vi "Module Loop.vi"(8 "error in (no error)":errorcluster, 11 "Sequencing in":refnum<class "Sequencing.lvclass">) -> (0 "error out":errorcluster, 3 "Sequencing out":refnum<class "Sequencing.lvclass">)   [LabVIEW 2020, in "VolatusSeq.lvlib" / "Sequencing.lvclass"]
uses:
  Sequencing.lvclass
  C:/dev/lv20CE/relink/lv-volatus/Volatus/Module/Module.lvclass
  Volatus/Module/Module.lvclass/Module.ctl
  Volatus/MessageQ/MessageQ.lvclass/MessageQ.ctl
  Sequencing.lvclass/Sequencing.ctl
  Volatus/Module/Module.lvclass
  Sequence Load Data.ctl
  lv-promises/Promises/Value/Value.lvclass
  Sequence Status.ctl
  Sequence Time.ctl
  Sequence Status Value/Sequence Status Value.lvclass/Sequence Status Value.ctl
  Sequence/Sequence.lvclass/Sequence.ctl
  Sequencing Status Value/Sequencing Status Value.lvclass/Sequencing Status Value.ctl
  lv-web-crypto/lv-crypto/Crypto/Hashes/SHA-256/SHA-256.lvclass
  d0d387a8-945a-4f27-bd1a-8c3fe56f864d.vi
  f3a44cdb-5a36-43f0-b83a-6d3fbfdadde6.vi
  31a4c29e-fb87-4ad3-ba8b-3d056e126c3f.vi
  93d0e60a-9556-42ac-a023-1725ae64f642.vi
  <vilib>/JDP Science/JSONtext/Next JSON Value.vi
  <vilib>/JDP Science/JSONtext/String Subset.vi
  Sequence/CRC.vi
  <vilib>/JDP Science/JSONtext/Parsing/Advance past next JSON Value (inlined COPY).vi
  <vilib>/JDP Science/JSONtext/Parsing/Advance past whitespace.vi
  <vilib>/JDP Science/JSONtext/Parsing/Advance past String.vi
  <vilib>/JDP Science/JSONtext/Parsing/Advance past Number.vi
  <vilib>/JDP Science/JSONtext/Parsing/Advance past Line Ending.vi
  <vilib>/JDP Science/JSONtext/Parsing/Parse Full Path or Item Name.vi
  <vilib>/JDP Science/JSONtext/Parsing/Advance past Array.vi
  <vilib>/JDP Science/JSONtext/Parsing/Advance past Object.vi
  <vilib>/JDP Science/JSONtext/support/Error Cluster From Code.vi
  <vilib>/JDP Science/JSONtext/Offset/Find Item Locations by Path.vi
  <vilib>/JDP Science/JSONtext/JSON text to Variant.vi
  <vilib>/JDP Science/JSONtext/LVClass Serializer/JSONtext LVClass Serializer.lvclass
  Sequence/Sequence.lvclass
  lv-promises/Promises/Promise/Promise.lvclass
  Sequence Status Value/Sequence Status Value.lvclass
  Sequencing Status Value/Sequencing Status Value.lvclass
  VolatusSeq.lvlib
  Volatus/MessageQ/MessageQ.lvclass
  <vilib>/JDP Science/JSONtext/JSONtext.lvlib
  lv-web-crypto/lv-crypto/Crypto/Crypto.lvlib
  C:/dev/lv20CE/relink/lv-volatus/VolatusSeq/Sequencing/Sequencing.lvclass
panel:
  out "Depth":i32
  in  "Abort":bool
  in  "Unload":bool
  in  "Start":bool
  in  "Load":bool
  in  "VSEQ":string="{\n    \"Sequence\": {\n        \"Name\": \"Bottle Condition\",\n        \"Version\": \"1\",\n        \"Comment\": \"Control state machine for bottle heating/cooling.\",\n        \"Entry\": \"Start\",\n        \"Abort\": \"Stop\",\n        \"States\": {\n            \"Start\": {\n                \"Comment\": \"Reset bottle controls to off state.\",\n                \"Steps\": [\n                    {\n                        \"Time\": 0,\n                        \"Commands\": [\n                            {\"Type\": \"Transition\", \"Target\": \"Hold\"}\n                        ]\n                    }\n                ]\n            },\n            \"Hold\": {\n                \"Comment\": \"Bottle in range, controls off.\",\n                \"Steps\": [\n                    {\n                        \"Time\": 0,\n                        \"Commands\": [\n                            {\"Type\": \"Digital\", \"Channel\": \"BottleCool\", \"Value\": false},\n                            {\"Type\": \"Digital\", \"Channel\": \"BottleHeat\", \"Value\": false}\n                        ]\n                    }\n                ],\n                \"Transitions\": [\n                    {\n                        \"Type\": \"State\",\n                        \"Target\": \"Cool\",\n                        \"Logic\": \"Any\",\n                        \"Conditions\": [\n                            {\"Type\": \"HighLimit\", \"Channel\": \"BottlePSI\", \"Limit\": 850}\n                        ]\n                    },\n                    {\n                        \"Type\": \"State\",\n                        \"Target\": \"Heat\",\n                        \"Logic\": \"Any\",\n                        \"Conditions\": [\n                            {\"Type\": \"LowLimit\", \"Channel\": \"BottlePSI\", \"Limit\": 750}\n                        ]\n                    }\n                ]\n            },\n            \"Cool\": {\n                \"Comment\": \"Cooling, wait for pressure to drop.\",\n                \"Steps\": [\n                    {\n                        \"Time\": 0,\n                        \"Commands\": [\n                            {\"Type\": \"Digital\", \"Channel\": \"BottleCool\", \"Value\": true}\n                        ]\n                    }\n                ],\n                \"Transitions\": [\n                    {\n                        \"Type\": \"State\",\n                        \"Target\": \"Start\",\n                        \"Logic\": \"Any\",\n                        \"Conditions\": [\n                            {\"Type\": \"LowLimit\", \"Channel\": \"BottlePSI\", \"Limit\": 800}\n                        ]\n                    }\n                ]\n            },\n            \"Heat\": {\n                \"Comment\": \"Heating, wait for pressure to rise.\",\n                \"Steps\": [\n                    {\n                        \"Time\": 0,\n                        \"Commands\": [\n                            {\"Type\": \"Digital\", \"Channel\": \"BottleHeat\", \"Value\": true}\n                        ]\n                    }\n                ],\n                \"Transitions\": [\n                    {\n                        \"Type\": \"State\",\n                        \"Target\": \"Start\",\n                        \"Logic\": \"Any\",\n                        \"Conditions\": [\n                            {\"Type\": \"HighLimit\", \"Channel\": \"BottlePSI\", \"Limit\": 800}\n                        ]\n                    }\n                ]\n            },\n            \"Stop\": {\n                \"Comment\": \"Stopping, ensure controls off.\",\n                \"Steps\": [\n                    {\n                        \"Time\": 0,\n                        \"Commands\": [\n                            {\"Type\": \"Digital\", \"Channel\": \"BottleCool\", \"Value\": false},\n                            {\"Type\": \"Digital\", \"Channel\": \"BottleHeat\", \"Value\": false}\n                        ]\n                    }\n                ]\n            }\n        }\n    }\n}"
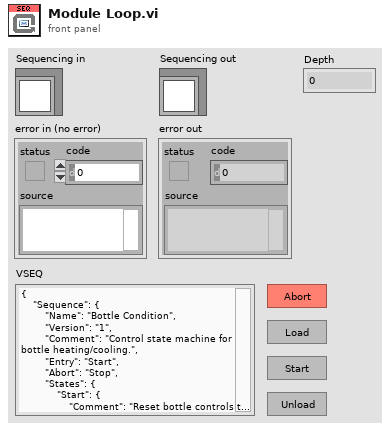
[diagram p1: front panel]
types:
  T1 = typedef "VolatusSeq.lvlib/Sequence Load Data.ctl" = cluster{"Name":string, "JSON":string, "Hash":string}
  T2 = enum32{"Invalid", "Standard", "Closed", "Hidden", "Minimized", "Maximized"}
  T3 = typedef "VolatusSeq.lvlib/Sequence Status.ctl" = cluster{"Name":string, "State":string, "Time":T4, "Running":bool, "Start Time":dbl, "Previous Duration":i64, "Previous Late":bool}
  T4 = typedef "VolatusSeq.lvlib/Sequence Time.ctl" = cluster{"Abort":bool, "Seq Time":dbl, "State Time":dbl, "Wall Time":dbl}
  T5 = typedef "VolatusSeq.lvlib/Sequencing Status.ctl" = cluster{"Sequences":T6[]}
  T6 = typedef "VolatusSeq.lvlib/Sequence Status Extended.ctl" = cluster{"Status":T3, "Loaded":bool, "CRC32":u32, "BG Color":string, "error":errorcluster}
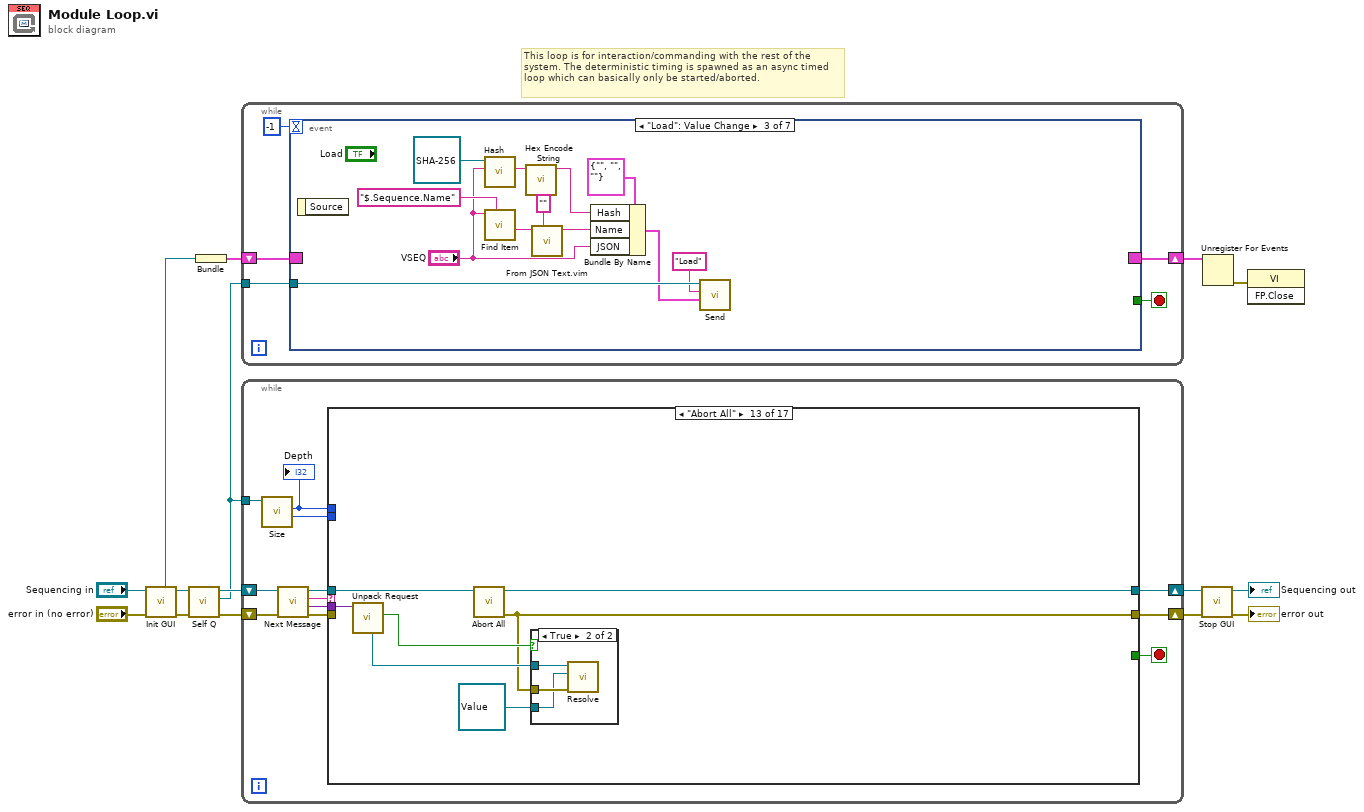
[diagram p0: block diagram]
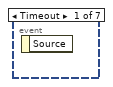
[diagram p2: hidden frame]
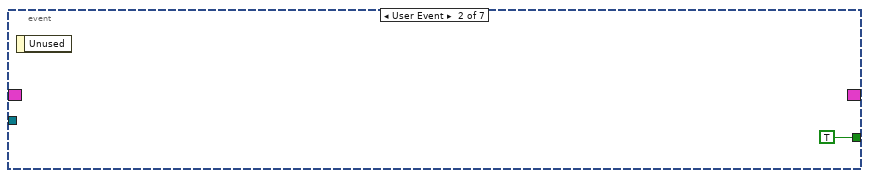
[diagram p3: hidden frame]
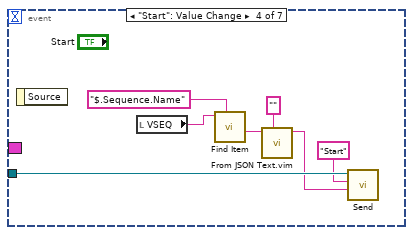
[diagram p4: hidden frame]
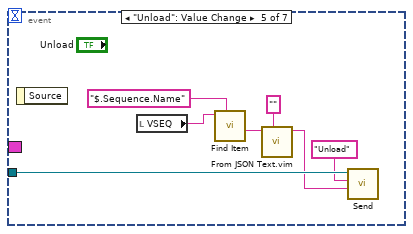
[diagram p5: hidden frame]
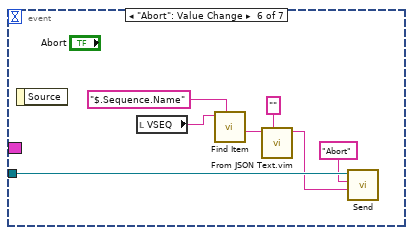
[diagram p6: hidden frame]
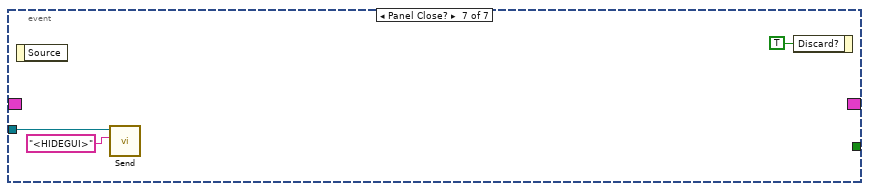
[diagram p7: hidden frame]
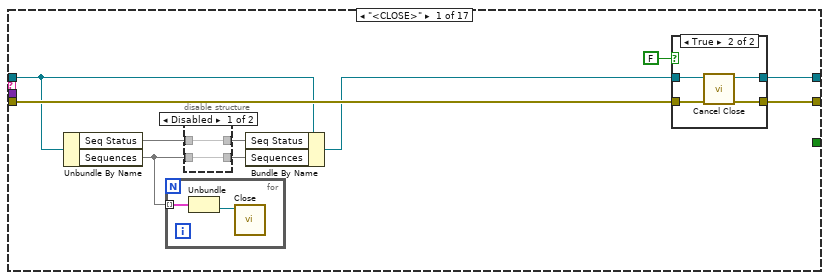
[diagram p8: hidden frame]
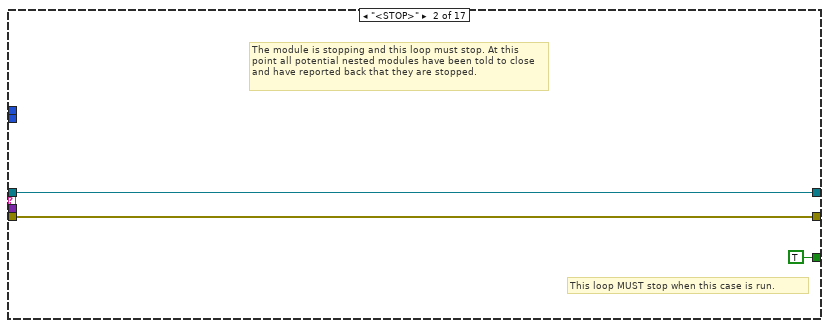
[diagram p11: hidden frame]
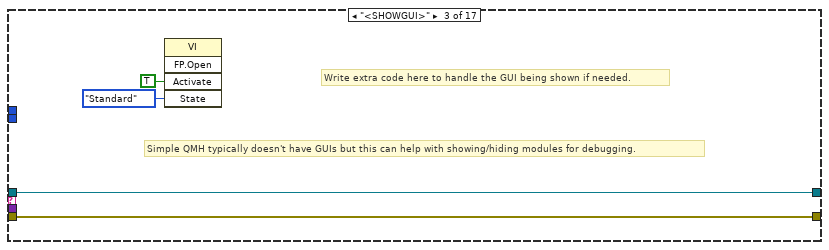
[diagram p12: hidden frame]
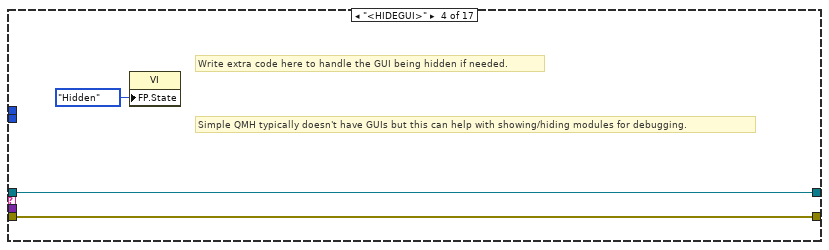
[diagram p13: hidden frame]
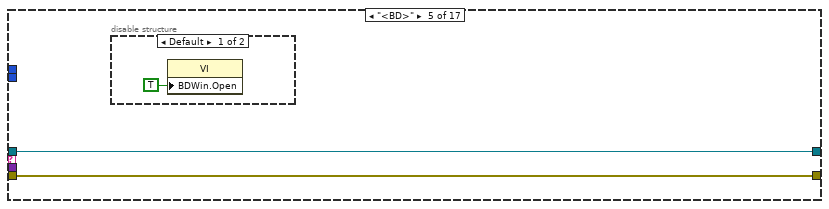
[diagram p14: hidden frame]
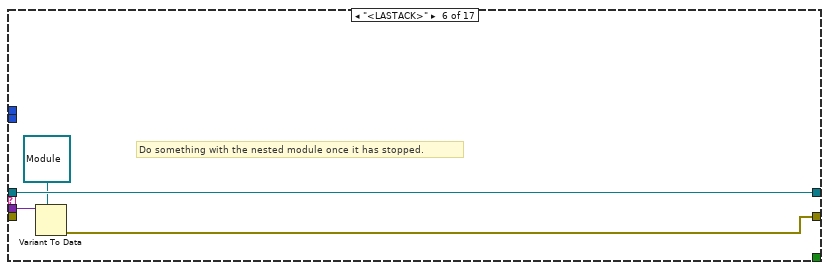
[diagram p16: hidden frame]
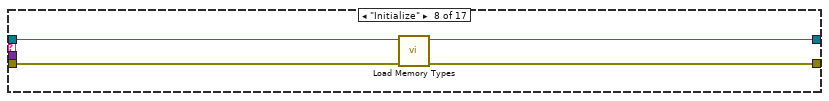
[diagram p18: hidden frame]
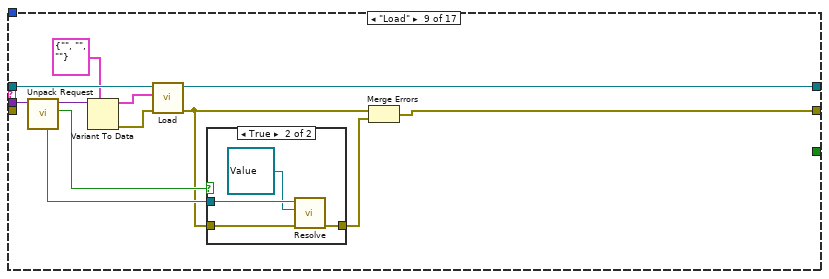
[diagram p19: hidden frame]
diagram:
  # "This loop is for interaction/commanding with the rest of the system. The deterministic timing is spawned as an async timed loop which can basically only be started/aborted."
  n1 = call "Init GUI.vi"("Module in"="Sequencing in") -> ("Module out"=w12:refnum<class "Sequencing.lvclass">, "Event Reg"=w10:refnum<event-registration>)  [unwired: 9 in]
  n2 = call "Self Q.vi"("Module in"=w12) -> ("Self Q"=w1:refnum<class "MessageQ.lvclass">, "Module out"=w8:refnum<class "Sequencing.lvclass">)  [unwired: 9 in]
  n3 = Bundle("Event Reg"=w10) -> (w11:cluster{"Event Reg":refnum<event-registration>})  [unwired: 1 in]
  n4 = while {
    tunnel: w1 -> [w18]
    shift-right: [w16] -> w4
    shift-left: w11 -> [w17]
    stop <- w15 stop-if-true
    n5 = event shown="[2] \"Load\": Value Change" {
      selector: w17 -> [_ _ _ _ _ _ _]
      dyn-events: [_ _ _ _ _ _ _] -> w16
      timeout: -1 -> [_ _ _ _ _ _ _]
      tunnel: w18 -> [_ _ w23 w34 w41 w48 w54]
      tunnel: [_ TRUE _ _ _ _ _] -> w15
      event Timeout {
        n6 = event-data() -> ()  [unwired: 1 in, 1 out]
      }
      event User Event {
        n7 = event-data() -> ()  [unwired: 1 in, 1 out]
      }
      event "Load": Value Change {
        n8 = event-data() -> ()  [unwired: 1 in, 1 out]
        n9 = call-dynamic "Hash.vi"("Message"="VSEQ", "SHA-256 in"=refnum<class "SHA-256.lvclass"> refnum) -> ("Hash"=w25:string)  [unwired: 7 in, 2 out]
        n10 = call <vilib>:"Find Item.vi"("$Path or Item Name"="$.Sequence.Name", "JSON"="VSEQ") -> ("<JSON>"=w30:string)  [unwired: 6 in, 3 out]
        n11 = call "Hex Encode String.vi"("String"=w25) -> ("Hex Encoded String"=w20:string)  [unwired: 10 in]
        n12 = call "From JSON Text.vim"("Data Type and Default Value"="", "JSON"=w30) -> ("Data out"=w26:string)  [unwired: 8 in, 1 out]
        n13 = Bundle By Name(cluster=T1 {"Name"="", "JSON"="", "Hash"=""} ("Sequence Load Data"), "Hash"=w20, "Name"=w26, "JSON"="VSEQ") -> (w22:T1)
        n14 = call "Send.vi"("Data"=w22, "ID"="Load", "MessageQ in"=w23) -> ()  [unwired: 7 in, 2 out]
      }
      event "Start": Value Change {
        n15 = event-data() -> ()  [unwired: 1 in, 1 out]
        n16 = local read "VSEQ"() -> (w35:string)
        n17 = call <vilib>:"Find Item.vi"("$Path or Item Name"="$.Sequence.Name", "JSON"=w35) -> ("<JSON>"=w37:string)  [unwired: 6 in, 3 out]
        n18 = call "From JSON Text.vim"("Data Type and Default Value"="", "JSON"=w37) -> ("Data out"=w33:string)  [unwired: 8 in, 1 out]
        n19 = call "Send.vi"("Data"=w33, "ID"="Start", "MessageQ in"=w34) -> ()  [unwired: 7 in, 2 out]
      }
      event "Unload": Value Change {
        n20 = event-data() -> ()  [unwired: 1 in, 1 out]
        n21 = local read "VSEQ"() -> (w42:string)
        n22 = call <vilib>:"Find Item.vi"("$Path or Item Name"="$.Sequence.Name", "JSON"=w42) -> ("<JSON>"=w44:string)  [unwired: 6 in, 3 out]
        n23 = call "From JSON Text.vim"("Data Type and Default Value"="", "JSON"=w44) -> ("Data out"=w40:string)  [unwired: 8 in, 1 out]
        n24 = call "Send.vi"("Data"=w40, "ID"="Unload", "MessageQ in"=w41) -> ()  [unwired: 7 in, 2 out]
      }
      event "Abort": Value Change {
        n25 = event-data() -> ()  [unwired: 1 in, 1 out]
        n26 = local read "VSEQ"() -> (w49:string)
        n27 = call <vilib>:"Find Item.vi"("$Path or Item Name"="$.Sequence.Name", "JSON"=w49) -> ("<JSON>"=w51:string)  [unwired: 6 in, 3 out]
        n28 = call "From JSON Text.vim"("Data Type and Default Value"="", "JSON"=w51) -> ("Data out"=w47:string)  [unwired: 8 in, 1 out]
        n29 = call "Send.vi"("Data"=w47, "ID"="Abort", "MessageQ in"=w48) -> ()  [unwired: 7 in, 2 out]
      }
      event Panel Close? {
        n30 = event-data() -> ()  [unwired: 1 in, 1 out]
        n31 = call "Send.vi"("ID"="<HIDEGUI>", "MessageQ in"=w54) -> ()  [unwired: 8 in, 2 out]
        n32 = event-data("Discard?"=TRUE) -> ()  [unwired: 1 in, 1 out]
      }
    }
  }
  n33 = while {
    shift-right: [w62] -> w5
    shift-left: w8 -> [w67]
    shift-right: [w61] -> w6
    shift-left: "error in (no error)" -> [w66]
    tunnel: w1 -> [w58]
    stop <- w60 stop-if-true
    n34 = call "Size.vi"("MessageQ in"=w58) -> ("Max Size"=w56:i32, "Depth"=w57:i32)  [unwired: 7 in, 2 out]
    "Depth" <- w57
    n35 = call "Next Message.vi"("error in (no error)"=w66, "Module in"=w67) -> ("error out"=w65:errorcluster, "Data"=w59:variant, "ID"=w64:string, "Module out"=w63:refnum<class "Sequencing.lvclass">)  [unwired: 6 in]
    n36 = case shown="\"Abort All\"" w64 {
      tunnel: w65 -> [w77 w89 w93 w96 w98 _ w105 w110 _ _ _ _ _ _ _ _ w231]
      tunnel: w63 -> [w70 w90 w94 w97 w99 w104 w106 w108 w122 w134 w148 w162 w174 w183 w207 w226 w229]
      tunnel: [w75 w90 w94 w97 w99 w104 w106 w107 w118 w133 w147 w161 w173 w181 w207 w225 w228] -> w62
      tunnel: [w76 w89 w93 w96 w98 w101 w105 w109 w111 w127 w141 w155 w169 w179 w201 w220 w230] -> w61
      tunnel: [_ TRUE _ _ _ _ _ _ _ _ _ _ _ _ _ _ _] -> w60
      tunnel: w59 -> [_ _ _ _ _ w103 _ _ w121 w137 w151 w165 w175 w185 w210 w224 _]
      tunnel: w57 -> [_ _ _ _ _ _ _ _ _ _ _ _ _ _ _ _ _]
      tunnel: w56 -> [_ _ _ _ _ _ _ _ _ _ _ _ _ _ _ _ _]
      frame "<CLOSE>" {
        n37 = Unbundle By Name(w70) -> ("Seq Status"=w68:map{string, T3}, "Sequences"=w73:map{string, refnum<class "Sequence.lvclass">})
        n38 = for {
          tunnel: w73 -> [w81] mode=indexing
          n39 = Unbundle(w81) -> ("Sequence"=w80:refnum<class "Sequence.lvclass">)  [unwired: 1 out]
          n40 = call "Close.vi"("Sequence in"=w80) -> ()  [unwired: 9 in, 2 out]
        }
        n41 = disable-structure shown="Disabled" {
          disable-tunnel: w73 -> [w79 _]
          disable-tunnel: [w79 _] -> w72
          disable-tunnel: [w78 _] -> w69
          disable-tunnel: w68 -> [w78 _]
          frame Disabled {
          }
          frame Enabled {
          }
        }
        n42 = Bundle By Name(cluster=w70, "Seq Status"=w69, "Sequences"=w72) -> (w71:refnum<class "Sequencing.lvclass">)
        n43 = case shown="True" FALSE {
          tunnel: w77 -> [w82 w87]
          tunnel: [w82 w86] -> w76
          tunnel: w71 -> [w83 w85]
          tunnel: [w83 w84] -> w75
          frame False {
          }
          frame True {
            n44 = call "Cancel Close.vi"("error in (no error)"=w87, "Module in"=w85) -> ("error out"=w86:errorcluster, "Module out"=w84:refnum<class "Sequencing.lvclass">)  [unwired: 8 in]
          }
        }
      }
      frame "<STOP>" {
        # "This loop MUST stop when this case is run."
        # "The module is stopping and this loop must stop. At this point all potential nested modules have been told to close and have reported back that they are stopped."
      }
      frame "<SHOWGUI>" {
        # "Simple QMH typically doesn't have GUIs but this can help with showing/hiding modules for debugging."
        # "Write extra code here to handle the GUI being shown if needed."
        n45 = invoke class="VI" method="FP.Open"("Activate"=TRUE ("Activate?"), "State"=T2."Standard") -> ()  [unwired: 3 in, 5 out]
      }
      frame "<HIDEGUI>" {
        # "Simple QMH typically doesn't have GUIs but this can help with showing/hiding modules for debugging."
        # "Write extra code here to handle the GUI being hidden if needed."
        n46 = property class="VI"("FP.State"=T2."Hidden" ("Front Panel Window:State")) -> ()  [unwired: 2 in, 2 out]
      }
      frame "<BD>" {
        n47 = disable-structure shown="Default" {
          frame condition #0 (active) {
            n48 = property class="VI"("BDWin.Open"=TRUE ("Block Diagram Window:Open")) -> ()  [unwired: 2 in, 2 out]
          }
          frame condition #1 {
          }
        }
      }
      frame "<LASTACK>" {
        # "Do something with the nested module once it has stopped."
        n49 = Variant To Data(type=refnum<class "Module.lvclass"> refnum ("Volatus:Module"), Variant=w103) -> (error out=w101:errorcluster)  [unwired: 1 in, 1 out]
      }
      frame "<TIMEOUT>" {
      }
      frame "Initialize" {
        n50 = call "Load Memory Types.vi"("error in (no error)"=w110, "Sequencing in"=w108) -> ("error out"=w109:errorcluster, "Sequencing out"=w107:refnum<class "Sequencing.lvclass">)  [unwired: 8 in]
      }
      frame "Load" {
        n51 = call "Unpack Request.vi"("Request Data"=w121) -> ("Is Request"=w115:bool, "Data"=w120:variant, "Promise"=w114:refnum<class "Promise.lvclass">)  [unwired: 8 in]
        n52 = Variant To Data(type=T1 {"Name"="", "JSON"="", "Hash"=""} ("Sequence Load Data"), Variant=w120) -> (data=w117:T1, error out=w116:errorcluster)  [unwired: 1 in]
        n53 = call "Load.vi"("error in (no error)"=w116, "Sequence Load Data"=w117, "Sequencing in"=w122) -> ("error out"=w113:errorcluster, "Sequencing out"=w118:refnum<class "Sequencing.lvclass">)  [unwired: 7 in]
        n54 = case shown="True" w115 {
          tunnel: w114 -> [_ w126]
          tunnel: w113 -> [_ w125]
          tunnel: [_ w124] -> w112
          frame False {
          }
          frame True {
            n55 = call "Resolve.vi"("error in (no error)"=w125, "Result (None)"=refnum<class "Value.lvclass"> refnum ("Result"), "Promise in"=w126) -> ("error out"=w124:errorcluster)  [unwired: 7 in, 1 out]
          }
        }
        n56 = Merge Errors(w113, w112) -> (w111:errorcluster)
      }
      frame "Start" {
        n57 = call "Unpack Request.vi"("Request Data"=w137) -> ("Is Request"=w131:bool, "Data"=w136:variant, "Promise"=w130:refnum<class "Promise.lvclass">)  [unwired: 8 in]
        n58 = Variant To Data(type="", Variant=w136) -> (data=w132:string, error out=w129:errorcluster)  [unwired: 1 in]
        n59 = call "Start.vi"("error in (no error)"=w129, "Sequence Name"=w132, "Sequencing in"=w134) -> ("error out"=w127:errorcluster, "Sequencing out"=w133:refnum<class "Sequencing.lvclass">)  [unwired: 7 in]
        n60 = case shown="True" w131 {
          tunnel: w130 -> [_ w140]
          tunnel: w127 -> [_ w139]
          tunnel: refnum<class "Value.lvclass"> refnum ("Result") -> [_ w138]
          frame False {
          }
          frame True {
            n61 = call "Resolve.vi"("error in (no error)"=w139, "Result (None)"=w138, "Promise in"=w140) -> ()  [unwired: 7 in, 2 out]
          }
        }
      }
      frame "Unload" {
        n62 = call "Unpack Request.vi"("Request Data"=w151) -> ("Is Request"=w145:bool, "Data"=w150:variant, "Promise"=w144:refnum<class "Promise.lvclass">)  [unwired: 8 in]
        n63 = Variant To Data(type="", Variant=w150) -> (data=w146:string, error out=w143:errorcluster)  [unwired: 1 in]
        n64 = call "Unload.vi"("error in (no error)"=w143, "Unload"=w146, "Sequencing in"=w148) -> ("error out"=w141:errorcluster, "Sequencing out"=w147:refnum<class "Sequencing.lvclass">)  [unwired: 7 in]
        n65 = case shown="True" w145 {
          tunnel: w144 -> [_ w154]
          tunnel: w141 -> [_ w153]
          tunnel: refnum<class "Value.lvclass"> refnum ("Result") -> [_ w152]
          frame False {
          }
          frame True {
            n66 = call "Resolve.vi"("error in (no error)"=w153, "Result (None)"=w152, "Promise in"=w154) -> ()  [unwired: 7 in, 2 out]
          }
        }
      }
      frame "Abort" {
        n67 = call "Unpack Request.vi"("Request Data"=w165) -> ("Is Request"=w159:bool, "Data"=w164:variant, "Promise"=w158:refnum<class "Promise.lvclass">)  [unwired: 8 in]
        n68 = Variant To Data(type="", Variant=w164) -> (data=w160:string, error out=w157:errorcluster)  [unwired: 1 in]
        n69 = call "Abort.vi"("error in (no error)"=w157, "Sequence Name"=w160, "Sequencing in"=w162) -> ("error out"=w155:errorcluster, "Sequencing out"=w161:refnum<class "Sequencing.lvclass">)  [unwired: 7 in]
        n70 = case shown="True" w159 {
          tunnel: w158 -> [_ w168]
          tunnel: w155 -> [_ w167]
          tunnel: refnum<class "Value.lvclass"> refnum ("Result") -> [_ w166]
          frame False {
          }
          frame True {
            n71 = call "Resolve.vi"("error in (no error)"=w167, "Result (None)"=w166, "Promise in"=w168) -> ()  [unwired: 7 in, 2 out]
          }
        }
      }
      frame "Abort All" {
        n72 = call "Unpack Request.vi"("Request Data"=w175) -> ("Is Request"=w172:bool, "Promise"=w171:refnum<class "Promise.lvclass">)  [unwired: 8 in, 1 out]
        n73 = call "Abort All.vi"("Sequencing in"=w174) -> ("error out"=w169:errorcluster, "Sequencing out"=w173:refnum<class "Sequencing.lvclass">)  [unwired: 9 in]
        n74 = case shown="True" w172 {
          tunnel: w171 -> [_ w178]
          tunnel: w169 -> [_ w177]
          tunnel: refnum<class "Value.lvclass"> refnum ("Result") -> [_ w176]
          frame False {
          }
          frame True {
            n75 = call "Resolve.vi"("error in (no error)"=w177, "Result (None)"=w176, "Promise in"=w178) -> ()  [unwired: 7 in, 2 out]
          }
        }
      }
      frame "Sequence Status" {
        n76 = Variant To Data(type=T3 {"Name"="", "State"="", "Time"={"Abort"=FALSE, "Seq Time"=0.0, "State Time"=0.0, "Wall Time"=0.0}, "Running"=FALSE, "Start Time"=0.0, "Previous Duration"=0, "Previous Late"=FALSE} ("Sequence Status"), Variant=w185) -> (data=w182:T3, error out=w180:errorcluster)  [unwired: 1 in]
        n77 = case shown="No Error" w180 {
          selector: w180 -> [_ w194]
          tunnel: w183 -> [w188 w193]
          tunnel: w182 -> [w187 _]
          tunnel: [w186 w193] -> w181
          tunnel: [_ w194] -> w179
          frame No Error {
            n78 = in-place {
              in-place-border: w187 -> [w189]
              n79 = in-place-cluster #1(w188) -> ("Seq Status"=w192:map{string, T3})
              n80 = Unbundle By Name(w189) -> ("Name"=w191:string)
              n81 = Insert Into Map(map in=w192, key=w191, value=w189) -> (map out=w190:map{string, T3})  [unwired: 2 out]
              n82 = in-place-cluster #1("Seq Status"=w190) -> (w186:refnum<class "Sequencing.lvclass">)
            }
          }
          frame Error {
          }
        }
      }
      frame "Request Seq Status" {
        # "Report error if sequence is unloaded."
        n83 = call "Unpack Request.vi"("Request Data"=w210) -> ("Data"=w209:variant, "Promise"=w203:refnum<class "Promise.lvclass">)  [unwired: 8 in, 1 out]
        n84 = Variant To Data(type="", Variant=w209) -> (data=w198:string, error out=w200:errorcluster)  [unwired: 1 in]
        n85 = Unbundle By Name(w207) -> ("Sequences"=w199:map{string, refnum<class "Sequence.lvclass">}, "Seq Status"=w206:map{string, T3})
        n86 = Look In Map(map=w199, key=w198) -> (key not found?=w195:bool)  [unwired: 1 in, 1 out]
        n87 = Look In Map(map=w206, key=w198) -> (key not found?=w197:bool, value=w205:T3)  [unwired: 1 in]
        n88 = Or(x=w195, y=w197) -> (x .or. y?=w196:bool)
        n89 = case shown="False" w196 {
          tunnel: w205 -> [w213 _]
          tunnel: [w212 _] -> w204
          tunnel: w198 -> [_ w217]
          tunnel: "Unknown sequence \"%s\"" -> [_ w216]
          tunnel: [_ w215] -> w211
          tunnel: w200 -> [_ w214]
          frame False {
            n90 = call "Create.vi"("Sequence Status"=w213) -> ("Sequence Status Value out"=w212:refnum<class "Sequence Status Value.lvclass">)  [unwired: 10 in]
          }
          frame True {
            n91 = Format Into String(format string=w216, w217) -> (resulting string=w219:string)  [unwired: 2 in, 1 out]
            n92 = call <vilib>:"Error Cluster From Error Code.vi"("error in (no error)"=w214, "error message (\"\")"=w219, "error code (0)"=15) -> ("error out"=w215:errorcluster)  [unwired: 6 in]
          }
        }
        n93 = call "Resolve.vi"("error in (no error)"=w211, "Result (None)"=w204, "Promise in"=w203) -> ("error out"=w201:errorcluster)  [unwired: 7 in, 1 out]
      }
      frame "Request Status" {
        n94 = call "Unpack Request.vi"("Request Data"=w224) -> ("Promise"=w223:refnum<class "Promise.lvclass">)  [unwired: 8 in, 2 out]
        n95 = call "Build Status.vi"("Sequencing in"=w226) -> ("error out"=w227:errorcluster, "Sequencing Status"=w222:T5, "Sequencing out"=w225:refnum<class "Sequencing.lvclass">)  [unwired: 8 in]
        n96 = call "Create.vi"("Status"=w222) -> ("Sequencing Status Value out"=w221:refnum<class "Sequencing Status Value.lvclass">)  [unwired: 10 in]
        n97 = call "Resolve.vi"("error in (no error)"=w227, "Result (None)"=w221, "Promise in"=w223) -> ("error out"=w220:errorcluster)  [unwired: 7 in, 1 out]
      }
      frame Default {
        n98 = call "Report Unhandled Message ID.vi"("error in (no error)"=w231, "Module in"=w229) -> ("error out"=w230:errorcluster, "Module out"=w228:refnum<class "Sequencing.lvclass">)  [unwired: 8 in]
      }
    }
  }
  n99 = call "Stop GUI.vi"("error in (no error)"=w6, "Module in"=w5) -> ("error out"=→"error out":errorcluster, "Module out"=→"Sequencing out":refnum<class "Sequencing.lvclass">)  [unwired: 8 in]
  n100 = Unregister For Events(event registration refnum=w4) -> (error out=w7:errorcluster)  [unwired: 1 in]
  n101 = invoke class="VI" method="FP.Close"(error in=w7) -> ()  [unwired: 2 in, 3 out]
